vi "Test Card Simulator Boolena text On Start.vi"(8 "error in (no error)":errorcluster, 11 "Test Case In":refnum<class "View Model Test.lvclass">) -> (0 "error out":errorcluster, 3 "Test Case Out":refnum<class "View Model Test.lvclass">)   [LabVIEW 2020, in "View Model Test.lvclass"]
uses:
  View Model Test.lvclass
  C:/Program Files (x86)/National Instruments/LabVIEW 2020/vi.lib/Astemes/LUnit/Test Case.lvclass
  ATM View Model/Controls.ctl
  ATM Controller/State.ctl
  <vilib>/Astemes/LUnit/Test Case.lvclass/Test Case.ctl
  01074fa8-ee8a-411d-bc8b-fc92c4f90959.vi
  <vilib>/Astemes/LUnit/Palette/Pass.vi
  <vilib>/Astemes/LUnit/Palette/Fail.vi
  <vilib>/Astemes/LUnit/Compare Variants.vi
  <vilib>/Astemes/LUnit/Describe Comparison.vi
  <vilib>/Astemes/LUnit/Set Assertion Type.vi
  <vilib>/Astemes/LUnit/Add test result.vi
  <vilib>/Astemes/LUnit/Variant to string.vi
  <vilib>/Astemes/LUnit/LUnit Record Assertion Result.vi
  <vilib>/Astemes/LUnit/LUnit Aggregate Assertion Results.vi
  <vilib>/Astemes/LUnit/Method Result/LUnit Merge Status.vi
  <vilib>/Astemes/LUnit/LUnit Concatenate result strings.vi
  <vilib>/Utility/Data Type/Get Type Information.vi
  <vilib>/Utility/LVClass/Get LV Class Name.vi
  View Model Test.lvclass/View Model Test.ctl
  ATM View Model/ATM View Model.lvclass
  ATM Controller/ATM Controller.lvclass
panel:
  out "Test Control":bool
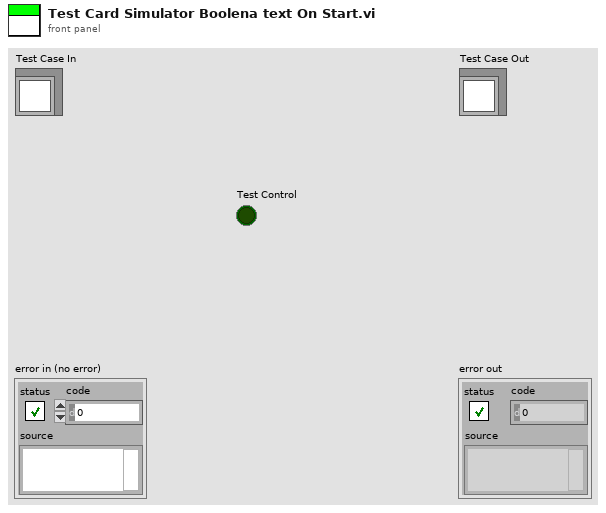
[diagram p1: front panel]
types:
  T1 = typedef "ATM Controller.lvclass/State.ctl" = enum16{"Start", "Card Inserted", "Verification Failed", "Verification Succeeded", "Depositing", "Depositing Completed", "Withdrawing", "Withdraw Completed", "Withdraw Failed", "Balance Inquiry", "Terminate"}
  T2 = typedef "ATM View Model.lvclass/Controls.ctl" = enum16{"User Input", "Enter", "Left Menu", "Right Menu", "Left Button", "Right Button", "Card Simulator"}
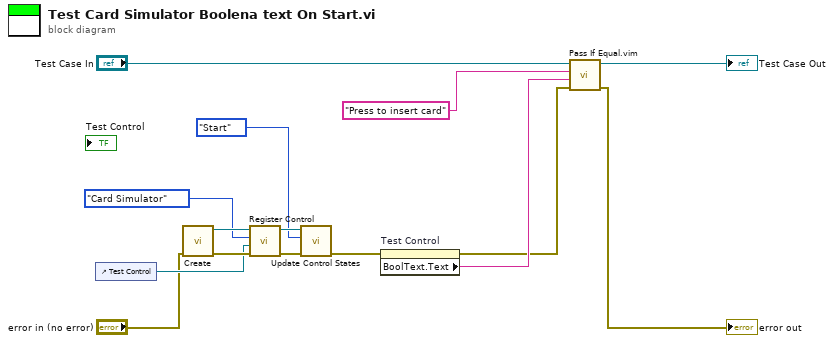
[diagram p0: block diagram]
diagram:
  n1 = control-ref of="Test Control"() -> (w8:refnum<vi>)
  n2 = call "Create.vi"("error in (no error)"="error in (no error)") -> ("error out"=w11:errorcluster, "ATM View Model out"=w12:refnum<class "ATM View Model.lvclass">)  [unwired: 9 in]
  n3 = call "Register Control.vi"("error in (no error)"=w11, "Control ref"=w8, "Control"=Controls."Card Simulator" ("Controls"), "ATM View Model in"=w12) -> ("error out"=w9:errorcluster, "ATM View Model out"=w10:refnum<class "ATM View Model.lvclass">)  [unwired: 6 in]
  n4 = call "Update Control States.vi"("error in (no error)"=w9, "ATM State"=State."Start", "ATM View Model In"=w10) -> ("error out"=w6:errorcluster)  [unwired: 7 in, 1 out]
  n5 = property on="Test Control" class="Bool (strict)"(error in=w6) -> (error out=w3:errorcluster, "BoolText.Text"=w5:string)  [unwired: 1 in, 1 out]
  n6 = call "Pass If Equal.vim"("error in (no error)"=w3, "Actual"=w5, "Expected"="Press to insert card" ("Boolean Text.Text"), "LUnit Test Case In"="Test Case In") -> ("error out"=→"error out":errorcluster, "LUnit Test Case Out"=→"Test Case Out":refnum<class "View Model Test.lvclass">)  [unwired: 6 in]
